vi "CC Observation Object to Script Command.vi"(8 "error in (no error)":errorcluster, 9 "Offsets":T3, 10 "RA and DEC String":cluster{"RA":string, "DEC":string}={"RA"="HH:MM:SS.nnn", "DEC"="DEG:arcmin:arcsec.nn"} caption="RA and DEC", 11 "Object.Name":string) -> (0 "error out":errorcluster, 2 "Object Name out":string, 3 "Define Object Step":T1={"Action"=enum."Acquire Images", "Data"=variant})   [LabVIEW 2024]
uses:
  Telescope/CC cluster Telescope Offsets.ctl
  typedefs/CC Script Step.ctl
  typedefs/CC enum Script Action.ctl
  typedefs/CC cluster Object.ctl
  typedefs/CC cluster sidereal rate.ctl
  typedefs/CC cluster RA and DEC.ctl
  typedefs/cc cluster muRA muDEC.ctl
  Telescope/Telescope cluster Equinox.ctl
  Telescope/Telescope cluster Parallax.ctl
  Telescope/Telescope cluster Rotator.ctl
  Telescope/Telesope ring Frame.ctl
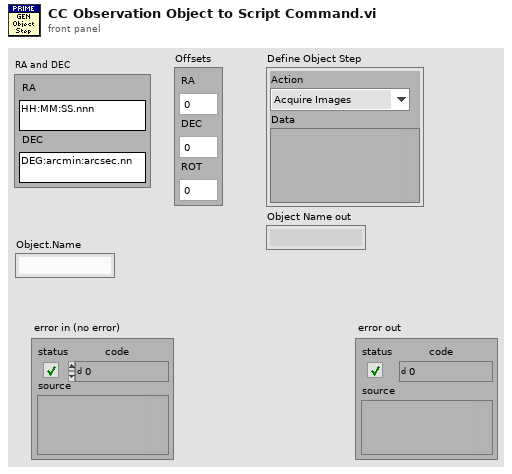
[diagram p1: front panel]
types:
  T1 = typedef "CC Script Step.ctl" = cluster{"Action":T2, "Data":variant}
  T2 = typedef "CC enum Script Action.ctl" = enum16{"Noop", "Define Object", "Define Exposure", "Define Dithering", "Acquire Images", "Set Filter Wheel", "Telescope Home", "Telescope Move", "Telescope RA DEC", "Focus Move Relative", "Focus Move Absolute", "Focus Set Home", "Macro", "Pause", "Ask User", "Define Random Dither", "CmdLine", "Outlet"}
  T3 = typedef "CC cluster Telescope Offsets.ctl" = cluster{"RA":dbl, "DEC":dbl, "ROT":dbl}
  T4 = typedef "CC cluster Object.ctl" = cluster{"Object":cluster{"Name":string}, "Sidereal Rate":T5, "RA and DEC":T6, "Proper Motion":T7, "Offsets":T3, "Equinox":T8, "Parallax":T9, "Rotator":T10, "Frame":T11, "Frac Rate":dbl, "Wavelength":dbl}
  T5 = typedef "CC cluster sidereal rate.ctl" = cluster{"dRA":dbl, "dDEC":dbl}
  T6 = typedef "CC cluster RA and DEC.ctl" = cluster{"RA":dbl, "DEC":dbl}
  T7 = typedef "cc cluster muRA muDEC.ctl" = cluster{"muRA":dbl, "muDEC":dbl, "Epoch":dbl}
  T8 = typedef "Telescope cluster Equinox.ctl" = cluster{"Equinox Year":i32, "Equinox Prefix":string}
  T9 = typedef "Telescope cluster Parallax.ctl" = cluster{"Parallax":dbl, "rv kps":dbl}
  T10 = typedef "Telescope cluster Rotator.ctl" = cluster{"Frame":string, "PA":dbl}
  T11 = typedef "Telesope ring Frame.ctl" = enum16{"FK4", "FK5", "APPT", "GAPPT", "AZEL"}
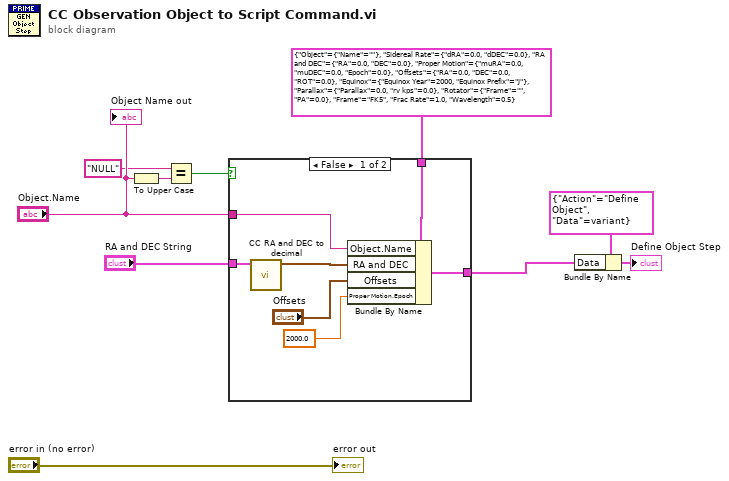
[diagram p0: block diagram]
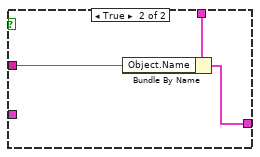
[diagram p2: hidden frame]
diagram:
  n1 = To Upper Case(1:"Object.Name") -> (0:w2:string)
  n2 = Equal?(x="NULL", y=w2) -> (x = y?=w1:bool)
  n3 = case shown="False" w1 {
    tunnel: T4 {"Object"={"Name"=""}, "Sidereal Rate"={"dRA"=0.0, "dDEC"=0.0}, "RA and DEC"={"RA"=0.0, "DEC"=0.0}, "Proper Motion"={"muRA"=0.0, "muDEC"=0.0, "Epoch"=0.0}, "Offsets"={"RA"=0.0, "DEC"=0.0, "ROT"=0.0}, "Equinox"={"Equinox Year"=2000, "Equinox Prefix"="J"}, "Parallax"={"Parallax"=0.0, "rv kps"=0.0}, "Rotator"={"Frame"="", "PA"=0.0}, "Frame"=enum."FK5", "Frac Rate"=1.0, "Wavelength"=0.5} ("Object") -> [w17 w20]
    tunnel: [w16 w18] -> w7
    tunnel: "RA and DEC String" -> [w15 _]
    tunnel: "Object.Name" -> [w11 w19]
    frame False {
      n4 = call "CC RA and DEC to decimal.vi"("RA and DEC String"=w15) -> ("RA and DEC"=w14:T6)  [unwired: 9 in, 1 out]
      n5 = Bundle By Name(cluster=w17, "Object.Name"=w11, "RA and DEC"=w14, "Offsets"="Offsets", "Proper Motion.Epoch"=2000.0 ("muRA muDEC Epoch.Epoch")) -> (w16:T4)
    }
    frame True {
      n6 = Bundle By Name(cluster=w20, "Object.Name"=w19) -> (w18:T4)
    }
  }
  n7 = Bundle By Name(cluster=T1 {"Action"=enum."Define Object", "Data"=variant} ("Cluster"), "Data"=w7) -> (→"Define Object Step":T1)
  "error out" <- "error in (no error)"
  "Object Name out" <- "Object.Name"
